vi "Read Max File Size.vi"(8 "error in (no error)":errorcluster, 11 "Error in":refnum<class "Error.lvclass">) -> (0 "error out":errorcluster, 2 "Max File Size":i64=10485760, 3 "Error out":refnum<class "Error.lvclass">)   [LabVIEW 2019, in "TSC Error.lvlib" / "Error.lvclass"]
uses:
  Error.lvclass
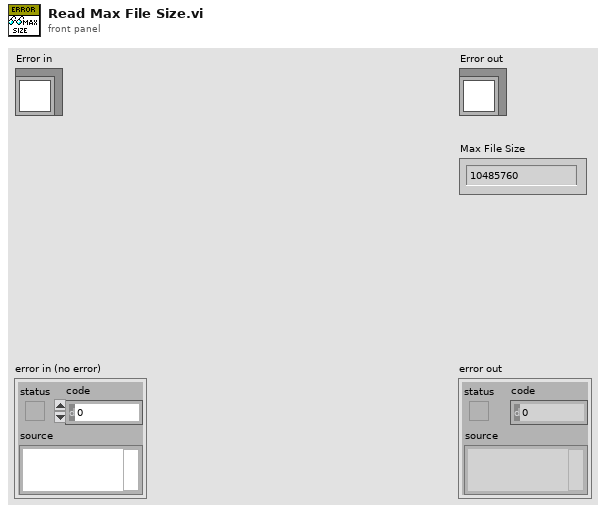
[diagram p1: front panel]
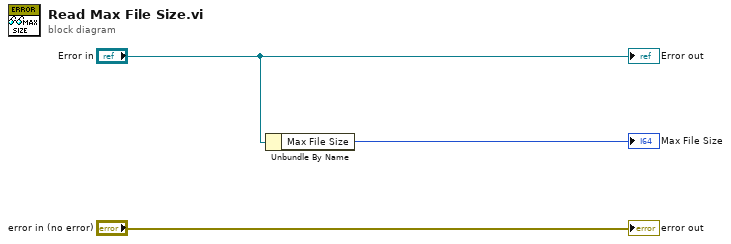
[diagram p0: block diagram]
diagram:
  n1 = Unbundle By Name("Error in") -> ("Max File Size"=→"Max File Size":i64)
  "error out" <- "error in (no error)"
  "Error out" <- "Error in"
